vi "fetch all records.vi"(0 "IVI Refnum in":refnum<k15>, 5 "error in (no error)":errorcluster, 7 "Channels":string, 9 "Time out":i32, 11 "Number of Records":i32) -> (4 "IVI Refnum out":refnum<k15>, 6 "error out":errorcluster, 14 "Records Done":i32, 15 "Fetched data":dbl[][](array[numeric]))   [LabVIEW 2014]
uses:
  <instrlib>/niScope/Acquire/Fetch/niScope Multi Fetch.vi
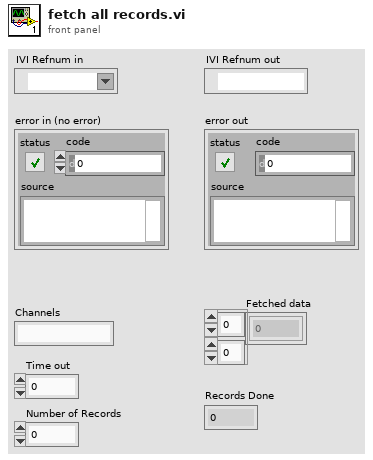
[diagram p1: front panel]
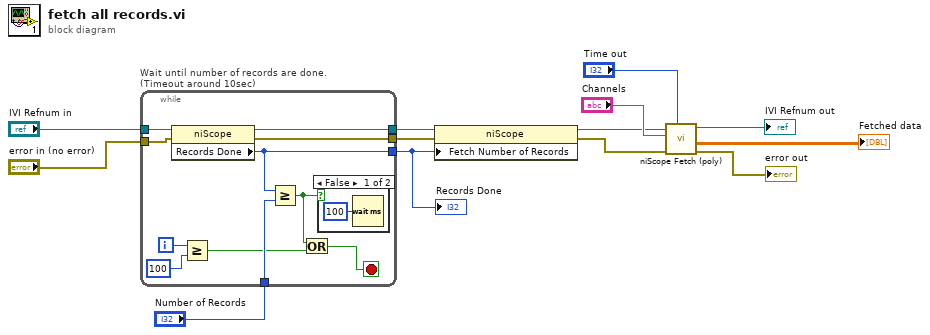
[diagram p0: block diagram]
diagram:
  n1 = while "Wait until number of records are done. (Timeout around 10sec)" {
    tunnel: "IVI Refnum in" -> [w24]
    tunnel: "error in (no error)" -> [w23]
    tunnel: [w22] -> w4
    tunnel: [w21] -> w3
    tunnel: [w20] -> w2
    tunnel: "Number of Records" -> [w19]
    i -> [w18]
    stop <- w15 stop-if-true
    n2 = property class="niScope"(reference=w24, error in=w23) -> (reference out=w22:refnum<k15>, error out=w21:errorcluster, "Records Done"=w20:i32)
    n3 = Greater Or Equal?(x=w18, y=100) -> (x >= y?=w16:bool)
    n4 = Greater Or Equal?(x=w20, y=w19) -> (x >= y?=w14:bool)
    n5 = Or(x=w14, y=w16) -> (x .or. y?=w15:bool)
    n6 = case shown="False" w14 {
      frame False {
        n7 = Wait (ms)(milliseconds to wait=u32 100) -> ()  [unwired: 1 out]
      }
      frame True {
      }
    }
  }
  "Records Done" <- w2
  n8 = property class="niScope"(reference=w4, error in=w3, "Fetch Number of Records"=w2) -> (reference out=w11:refnum<k15>, error out=w12:errorcluster)
  n9 = call-poly <instrlib>:"niScope Fetch (poly).vi"("timeout"="Time out", "error in"=w12, "channels"="Channels", "instrument handle"=w11) -> ("error out"=→"error out":errorcluster, "wfm"=→"Fetched data":dbl[][], "instrument handle out"=→"IVI Refnum out":refnum<k15>)  [unwired: 4 in, 1 out]
